vi "Initialise.vi"(7 "Oriel (custom drivers)":T1, 8 "error in (no error)":errorcluster) -> (0 "error out":errorcluster, 1 "Mono Connected?":bool, 5 "Oriel (custom drivers) out":T1)   [LabVIEW 2017, in "Monochromator.lvlib" / "Oriel (custom drivers).lvlib"]
uses:
  Oriel (custom drivers).lvlib
  Controls/Params.ctl
  D:/Optical Software Code V1.6/Optical Software Code/Modules/Monochromator/Cornerstone.dll
  Cornerstone.dll
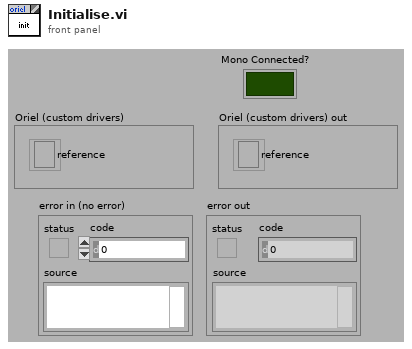
[diagram p1: front panel]
types:
  T1 = typedef "Monochromator.lvlib/Oriel (custom drivers).lvlib/Params.ctl" = cluster{"reference":refnum<k24>}
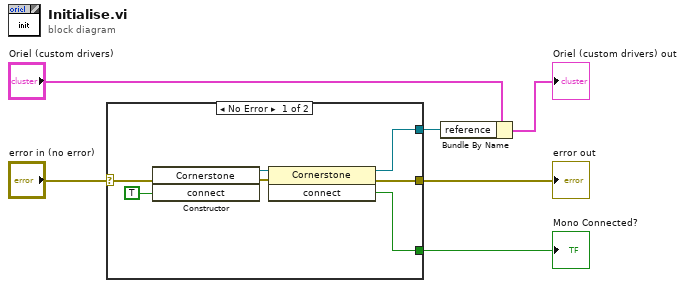
[diagram p0: block diagram]
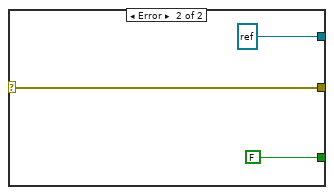
[diagram p2: hidden frame]
diagram:
  n1 = case shown="No Error" "error in (no error)" {
    selector: "error in (no error)" -> [w13 w16]
    tunnel: [w8 w16] -> w5
    tunnel: [w9 FALSE] -> w4
    tunnel: [w7 refnum<k24> refnum ("new reference")] -> w1
    frame No Error {
      n2 = constructor class="Cornerstone"(error in=w13, "connect"=TRUE) -> (reference out=w11:refnum<k24>, error out=w10:errorcluster)  [unwired: 2 in, 2 out]
      n3 = invoke class="Cornerstone" method="connect"(reference=w11, error in=w10) -> (reference out=w7:refnum<k24>, error out=w8:errorcluster, "connect"=w9:bool)  [unwired: 1 in]
    }
    frame Error {
    }
  }
  "error out" <- w5
  "Mono Connected?" <- w4
  n4 = Bundle By Name(cluster="Oriel (custom drivers)", "reference"=w1) -> (→"Oriel (custom drivers) out":T1)
